vi "hsdcWriteToDRAM_7975.vi"(6 "inputValid":bool, 8 "start":bool, 10 "hsdcPoints":u32, 11 "input":i16) -> (3 "hsdcRunning":bool)   [LabVIEW 2016]
uses:
  <vilib>/rvi/Memory/Memory_Emulation/niFpgaMemoryFastEmulationDramWriteAndRequestData.vi
  <vilib>/rvi/Memory/Memory_Emulation/niFpgaMemoryEmulationDramWriteAndRequestData.vi
  <vilib>/rvi/DataTransferAndStorage/Container/Common/niFpgaContainerGetUniqueNameForEmu.vi
  <vilib>/rvi/Memory/Memory_Emulation/niFpgaMemoryEmulationDramWriteAndRequestDataApplyByteEnables.vi
  <vilib>/rvi/DataTransferAndStorage/Container/XNode/niFpgaContainer.xnode
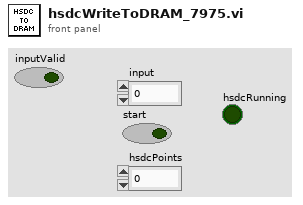
[diagram p1: front panel]
types:
  T1 = cluster{"Element 1":i16, "Element 2":i16, "Element 3":i16, "Element 4":i16}
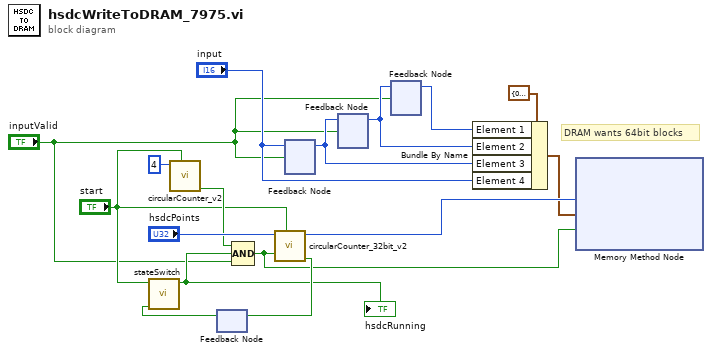
[diagram p0: block diagram]
diagram:
  # "DRAM wants 64bit blocks"
  n1 = call "circularCounter_v2.vi"("reset"="start", "maxCount"=u16 4) -> ("maxReached"=w9:bool)  [unwired: 6 in, 3 out]
  n2 = feedback #1() -> (w16:bool)  [unwired: 1 in]
  n3 = call "stateSwitch.vi"("disable"=w16, "enable"="start") -> ("state"=w4:bool)  [unwired: 9 in]
  "hsdcRunning" <- w4
  n4 = Compound Arithmetic op=AND(w9, w4, "inputValid") -> (w5:bool)
  n5 = call "circularCounter_32bit_v2.vi"("reset"="start", "doStep"=w5, "maxCount"="hsdcPoints") -> ("maxReached"=w15:bool, "index"=w13:u32)  [unwired: 5 in, 2 out]
  n6 = feedback-in #1(w15) -> ()
  n7 = feedback #2() -> (w8:i16)  [unwired: 1 in]
  n8 = feedback-in #2("input", "inputValid") -> ()
  n9 = feedback #3() -> (w7:i16)  [unwired: 1 in]
  n10 = feedback-in #3(w8, "inputValid") -> ()
  n11 = feedback #4() -> (w6:i16)  [unwired: 1 in]
  n12 = feedback-in #4(w7, "inputValid") -> ()
  n13 = Bundle By Name(cluster=T1 {"Element 1"=0, "Element 2"=0, "Element 3"=0, "Element 4"=0} ("dram_4xI16"), "Element 1"=w6, "Element 2"=w7, "Element 3"=w8, "Element 4"="input") -> (w11:T1)
  n14 = xnode ("Memory Method Node")("Address"=w13, "Data"=w11, "Input Valid"=w5) -> ()  [unwired: 1 in, 2 out]
